vi "Mod_OFDM_Get_Data_Sources.vi"(0 "Configuration in":variant, 11 "error in":errorcluster) -> (2 "# of Data Sources":i32, 3 "Initial SEED IN":u32[](array[numeric]), 4 "Configuration out":variant, 6 "Attribute Name":string, 8 "Pool of Data Sources":T1 {"Register Initial State" format="%08x"}, 10 "Data Source Names":string[](array[string]), 15 "error out":errorcluster)   [LabVIEW 2010]
doc: "The VI retrieves the attribute value for the data sources. The data sources is an array of clusters. Each cluster represents a unique data source. This forms the pool of Data sources with which the OFDM frame is configured."
uses:
  Controls(Type_DEf)/Attribute Data Types.ctl
  Controls(Type_DEf)/Configure Pulse Shaping.ctl
  Controls(Type_DEf)/Pool of Modulator Control.ctl
  Controls(Type_DEf)/Pool of Data Source Control.ctl
  Controls(Type_DEf)/Attribute Names.ctl
panel:
  in  "Attribute Data Types":T2={"Pulse Shaping"={"System Filter"={"TX Filter"=enum."none", "Alpha"=0.0, "filter length"=0}, "Modulation system parameters"={"samples per symbol (16)"=0}, "symbol rate (Hz)"=0.0}, "FRAME Table"=[], "OFDM Frame"=[], "Sub Carrier Selection"={"Sub Carrier Selection"=[], "OFDM Parameters"={"# of Sub Carrier"=0, "Length Of Cylic Prefix"=0}}, "Symbol Table"=[], "Symbol Pool"=[], "Pool of Modulators"=[], "Pool of Data Sources"=[], "Atribute Names"={"Data Source Pool"="Data Source Pool ", "Modulator Source Pool"="Modulator Source Pool ", "OFDM SYMBOL POOL"="OFDM SYMBOL POOL", "Symbol Table"="Symbol Table", "Sub Carrier Selection"="Sub Carrier Selection", "OFDM Frame"="OFDM Frame", "FRAME Table"="FRAME Table", "Pulse Shaping"="Pulse Shaping"}} {"Pool of Data Sources"."Register Initial State" format="%08x"; "Pulse Shaping"."symbol rate (Hz)" min=1.0 step=1.0 format="%.2p"; "Pulse Shaping"."Modulation system parameters"."samples per symbol (16)" step=2; "Pulse Shaping"."System Filter"."Alpha" min=0.0 max=1.0 step=0.05 format="%.2f"}
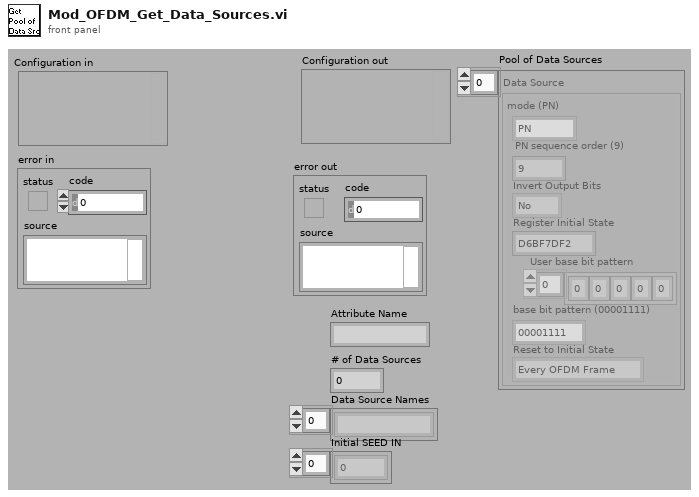
[diagram p1: front panel]
types:
  T1 = typedef "Pool of Data Source Control.ctl" = cluster{"mode (PN)":enum16{"PN", "pattern", "user"}, "PN sequence order (9)":i32, "Invert Output Bits":enum16{"No", "Yes"}, "Register Initial State ":u32, "User base bit pattern":i8[], "base bit pattern (00001111)":enum16{"0", "1", "01", "0011", "00001111"}, "Reset to Initial State":enum16{"Every OFDM Frame", "Every OFDM Symbol", "Every Sub Carrier"}}[]
  T2 = typedef "Attribute Data Types.ctl" = cluster{"Pulse Shaping":T3, "FRAME Table":string[][], "OFDM Frame":cluster{"Symbol Name":string, "# of Symbols":i32}[], "Sub Carrier Selection":cluster{"Sub Carrier Selection":cluster{"Sub Carrier":bool, "Data Source":u16, "Modulator":u16}[], "OFDM Parameters":cluster{"# of Sub Carrier":i32, "Length Of Cylic Prefix":i32}}, "Symbol Table":string[][], "Symbol Pool":string[], "Pool of Modulators":T4, "Pool of Data Sources":T1, "Atribute Names":T5}
  T3 = typedef "Configure Pulse Shaping.ctl" = cluster{"System Filter":cluster{"TX Filter":enum16{"none", "Raised Cosine", "Root Raised Cos"}, "Alpha":dbl, "filter length":i32}, "Modulation system parameters":cluster{"samples per symbol (16)":u32}, "symbol rate (Hz)":dbl}
  T4 = typedef "Pool of Modulator Control.ctl" = cluster{"M-QAM":enum16{"4", "16", "64", "256"}, "M-PSK":enum16{"2", "4", "8", "16", "32", "64", "128", "256"}, "Type of Modulation":enum16{"PSK", "QAM"}, " PSK":cluster{"differential PSK":enum16{"disable", "enable"}, "PSK type":enum16{"normal", "shifted", "offset"}}}[]
  T5 = typedef "Attribute Names.ctl" = cluster{"Data Source Pool":string, "Modulator Source Pool":string, "OFDM SYMBOL POOL":string, "Symbol Table":string, "Sub Carrier Selection":string, "OFDM Frame":string, "FRAME Table":string, "Pulse Shaping":string}
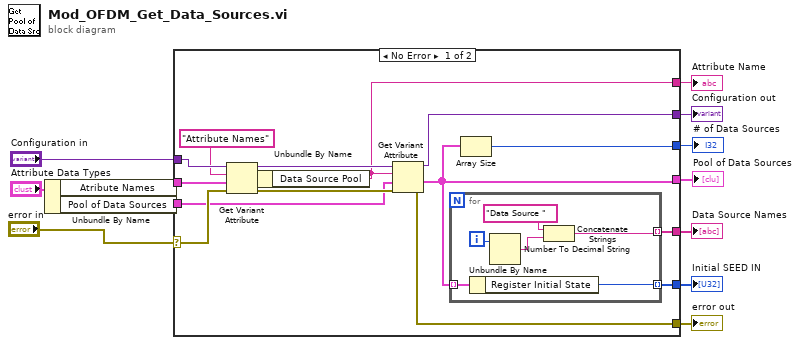
[diagram p0: block diagram]
diagram:
  n1 = Unbundle By Name("Attribute Data Types") -> ("Atribute Names"=w6:T5, "Pool of Data Sources"=w5:T1)
  n2 = case shown="No Error" "error in" {
    selector: "error in" -> [w24 w34]
    tunnel: [w27 w34] -> w11
    tunnel: "Configuration in" -> [w20 _]
    tunnel: [w26 _] -> w9
    tunnel: [w15 _] -> w8
    tunnel: w6 -> [w22 _]
    tunnel: w5 -> [w23 _]
    tunnel: [w17 _] -> w4
    tunnel: [w16 _] -> w3
    tunnel: [w14 _] -> w2
    tunnel: [w13 _] -> w1
    frame No Error {
      n3 = Get Variant Attribute(Variant=w20, name="Attribute Names", default value (empty Variant)=w22, error in=w24) -> (duplicate Variant=w21:variant, value=w18:T5, error out=w25:errorcluster)  [unwired: 1 out]
      n4 = Unbundle By Name(w18) -> ("Data Source Pool"=w16:string)
      n5 = Get Variant Attribute(Variant=w21, name=w16, default value (empty Variant)=w23, error in=w25) -> (duplicate Variant=w26:variant, value=w15:T1, error out=w27:errorcluster)  [unwired: 1 out]
      n6 = for {
        tunnel: [w30] -> w17 mode=indexing
        tunnel: w15 -> [w29] mode=indexing
        tunnel: [w28] -> w13 mode=indexing
        i -> [w33]
        n7 = Unbundle By Name(w29) -> ("Register Initial State"=w28:u32)
        n8 = Number To Decimal String(number=w33) -> (decimal integer string=w32:string)  [unwired: 1 in]
        n9 = Concatenate Strings("Data Source " ("string"), w32) -> (w30:string)
      }
      n10 = Array Size(array=w15) -> (size(s)=w14:i32)
    }
    frame Error {
    }
  }
  "error out" <- w11
  "Configuration out" <- w9
  "Pool of Data Sources" <- w8
  "Data Source Names" <- w4
  "Attribute Name" <- w3
  "# of Data Sources" <- w2
  "Initial SEED IN" <- w1
